vi "getFirstPixelPos.vi"(8 "error in (no error)":errorcluster, 10 "Cluster":T1, 11 "Cam 0":T2) -> (0 "error out":errorcluster, 1 "first Pixel position":dbl, 2 "Cluster out":T1, 3 "Cam out":T2)   [LabVIEW 2013]
uses:
  configTypDEf.ctl
  CamSettingSUB_TypDEf.ctl
  CamAndObj_TypDEf.ctl
  shared/OnOffTypeDef.ctl
  userROI.ctl
  shared/numericVariable_TypeDef.ctl
  CamRoiTypDef.ctl
  BaseDriver/BaseDriver.lvclass
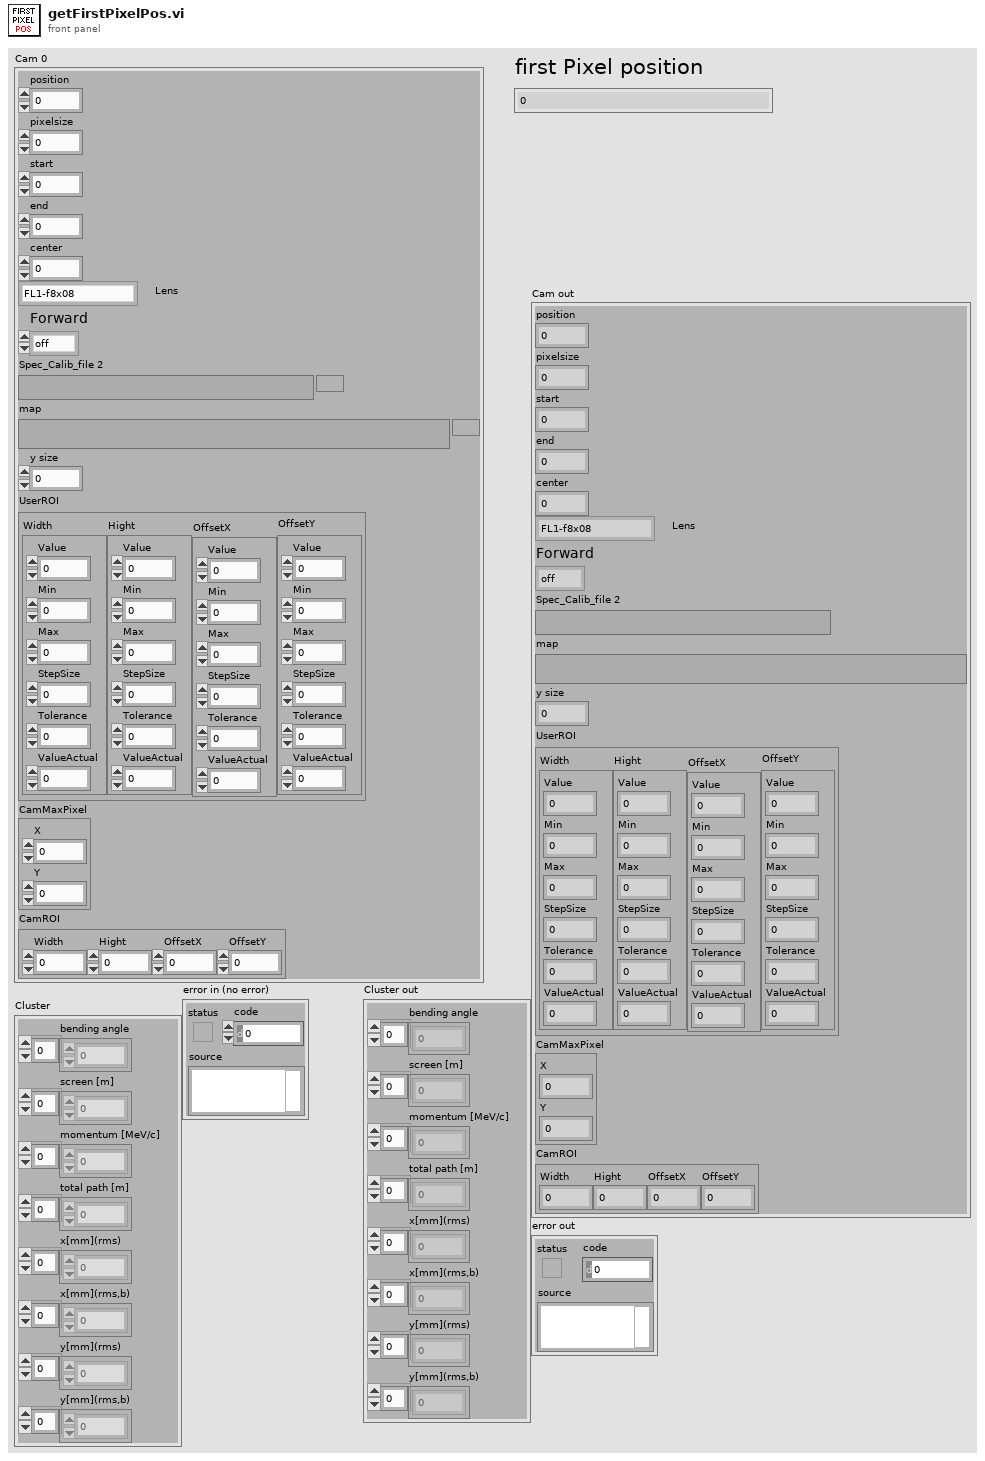
[diagram p1: front panel]
types:
  T1 = typedef "configTypDEf.ctl" = cluster{"bending angle":dbl[], "screen [m]":dbl[], "momentum [MeV/c]":dbl[], "total path [m]":dbl[], "x[mm](rms)":dbl[], "x[mm](rms,b)":dbl[], "y[mm](rms)":dbl[], "y[mm](rms,b)":dbl[]}
  T2 = typedef "CamSettingSUB_TypDEf.ctl" = cluster{"position":dbl, "pixelsize":dbl, "start":dbl, "end":dbl, "center":dbl, "Lens":T3, "Forward":T4, "Spec_Calib_file 2":path, "map":path, "y size":i32, "UserROI":T5, "CamMaxPixel":cluster{"X":i32, "Y":i32}, "CamROI":T7}
  T3 = typedef "CamAndObj_TypDEf.ctl" = enum16{"FL1-f8x08", "FL1-f8x06", "FL1-f8", "ch300-f50", "FL2G-f8", "FL3M14-f8", "FL3M14-f8x08", "FL3M14-f8x08(2x2)"}
  T4 = typedef "OnOffTypeDef.ctl" = enum16{"off", "on"}
  T5 = typedef "userROI.ctl" = cluster{"Width":T6, "Hight":T6, "OffsetX":T6, "OffsetY":T6}
  T6 = typedef "BaseDriver.lvclass/numericVariable_TypeDef.ctl" = cluster{"Value":dbl, "Min":dbl, "Max":dbl, "StepSize":dbl, "Tolerance":dbl, "ValueActual":dbl}
  T7 = typedef "CamRoiTypDef.ctl" = cluster{"Width":dbl, "Hight":dbl, "OffsetX":dbl, "OffsetY":dbl}
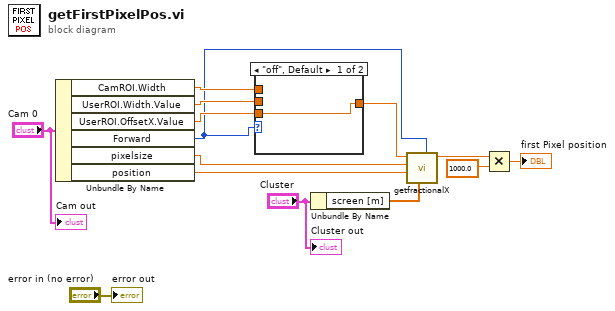
[diagram p0: block diagram]
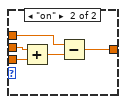
[diagram p2: hidden frame]
diagram:
  n1 = Unbundle By Name("Cam 0") -> ("CamROI.Width"=w3:dbl, "UserROI.Width.Value"=w4:dbl, "UserROI.OffsetX.Value"=w5:dbl, "Forward"=w1:T4, "pixelsize"=w8:dbl, "position"=w9:dbl)
  n2 = case shown="\"off\", Default" w1 {
    tunnel: w5 -> [w15 w20]
    tunnel: w4 -> [_ w19]
    tunnel: w3 -> [_ w18]
    tunnel: [w15 w16] -> w2
    frame "off", Default {
    }
    frame "on" {
      n3 = Add(x=w19, y=w20) -> (x+y=w17:dbl)
      n4 = Subtract(x=w18, y=w17) -> (x-y=w16:dbl)
    }
  }
  n5 = Unbundle By Name("Cluster") -> ("screen [m]"=w11:dbl[])
  n6 = call "getfractionalX.vi"("forward"=w1, "screen [m]"=w11, "position"=w9, "pixelsize"=w8, "Numeric in"=w2) -> ("position m"=w12:dbl)  [unwired: 5 in, 1 out]
  n7 = Multiply(x=w12, y=1000.0) -> (x*y=→"first Pixel position":dbl)
  "Cam out" <- "Cam 0"
  "Cluster out" <- "Cluster"
  "error out" <- "error in (no error)"
